vi "Set Output Node Linkage.vi"(7 "Add?":bool, 8 "error in":errorcluster, 11 "Section Ref in":T1 format="%.0x") -> (0 "error out":errorcluster, 3 "Item Ref out":T1 format="%.0x")   [LabVIEW 2019, in "Control Addon Shared.lvlib"]
uses:
  Control Addon Shared.lvlib
  <vilib>/NI VeriStand/Custom Device API/Custom Device Item Ref.ctl
  NationalInstruments.VeriStand.SystemStorage
  Constants.vi
  <vilib>/NI/NI VeriStand Advanced SysDef API/_SubVIs/SysDef.Search.GUID.vi
  <vilib>/NI/NI VeriStand Advanced SysDef API/_SubVIs/SysDef.Property.Get.Node.vi
  <vilib>/NI/NI VeriStand Advanced SysDef API/SysDef API/Advanced System Definition.lvlib
  <vilib>/NI VeriStand/Custom Device API/Custom Device API.lvlib
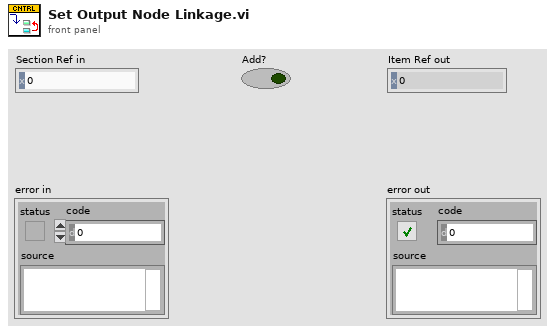
[diagram p1: front panel]
types:
  T1 = typedef "Custom Device API.lvlib/Custom Device Item Ref.ctl" = u64
  T2 = typedef "Custom Device API.lvlib/Custom Device Pointer.ctl" = refnum<k24>
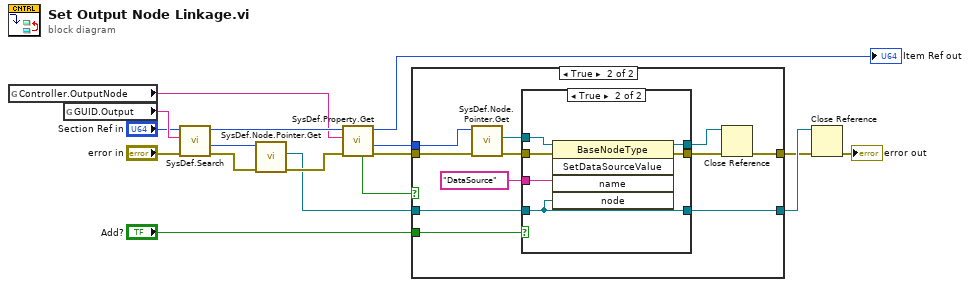
[diagram p0: block diagram]
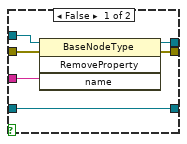
[diagram p3: hidden frame]
diagram:
  n1 = global read "Constants.vi" "Controller.OutputNode"() -> (w7:string)
  n2 = global read "Constants.vi" "GUID.Output"() -> (w15:string)
  n3 = call-poly <vilib>:"SysDef.Search.vi"("error in (no error)"="error in", "GUID"=w15, "nodeID"="Section Ref in") -> ("error out"=w4:errorcluster, "Value out"=w3:u64, "nodeID out"=w14:u64)  [unwired: 5 in, 1 out]
  n4 = call <vilib>:"SysDef.Node.Pointer.Get.vi"("error in (no error)"=w4, "nodeID"=w3) -> ("error out"=w2:errorcluster, "Node Pointer"=w1:T2)  [unwired: 6 in, 2 out]
  n5 = call-poly <vilib>:"SysDef.Property.Get.vi"("error in (no error)"=w2, "Property Name"=w7, "nodeID"=w14) -> ("error out"=w16:errorcluster, "Value out"=w17:u64, "nodeID out"=→"Item Ref out":u64, "Found?"=w6:bool)  [unwired: 5 in]
  n6 = case shown="False" w6 {
    tunnel: w17 -> [_ w23]
    tunnel: w16 -> [w18 w21]
    tunnel: w1 -> [w19 w29]
    tunnel: [w18 w26] -> w5
    tunnel: [w19 w28] -> w13
    tunnel: "Add?" -> [_ w27]
    frame False {
    }
    frame True {
      n7 = call <vilib>:"SysDef.Node.Pointer.Get.vi"("error in (no error)"=w21, "nodeID"=w23) -> ("error out"=w20:errorcluster, "Node Pointer"=w22:T2)  [unwired: 6 in, 2 out]
      n8 = case shown="True" w27 {
        tunnel: [w33 w42] -> w24
        tunnel: [w34 w41] -> w25
        tunnel: w29 -> [w31 w37]
        tunnel: w20 -> [w35 w40]
        tunnel: w22 -> [w36 w39]
        tunnel: "DataSource" ("name") -> [w32 w38]
        tunnel: [w31 w37] -> w28
        frame False {
          n9 = invoke class="BaseNodeType" method="RemoveProperty"(reference=w36, error in=w35, "name"=w32) -> (reference out=w33:T2, error out=w34:errorcluster)  [unwired: 1 in, 2 out]
        }
        frame True {
          n10 = invoke class="BaseNodeType" method="SetDataSourceValue"(reference=w39, error in=w40, "name"=w38, "node"=w37) -> (reference out=w42:T2, error out=w41:errorcluster)  [unwired: 1 in, 3 out]
        }
      }
      n11 = Close Reference(reference=w24, error in (no error)=w25) -> (error out=w26:errorcluster)
    }
  }
  n12 = Close Reference(reference=w13, error in (no error)=w5) -> (error out=→"error out":errorcluster)
